vi "myRIO_BRig_RT_dataExp_BUR_min.vi"() -> (2 "output_BUR_min":i32)   [LabVIEW 2014]
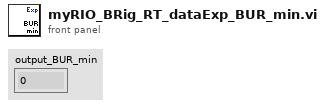
[diagram p1: front panel]
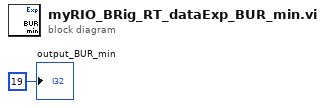
[diagram p0: block diagram]
diagram:
  "output_BUR_min" <- 19 ("output_iBlock")
